vi "Get Full Tree.vi"(8 "error in (no error)":errorcluster, 11 "OpenHW in":refnum<class "OpenHW.lvclass">) -> (0 "error out":errorcluster, 2 "Full Tree":T1[](array[typedef]), 3 "OpenHW out":refnum<class "OpenHW.lvclass">)   [LabVIEW 2022 SP3, in "open-hw-mon-lv.lvlib" / "OpenHW.lvclass"]
uses:
  OpenHW.lvclass
  OpenHW.lvclass/OpenHW.ctl
  HW Node.ctl
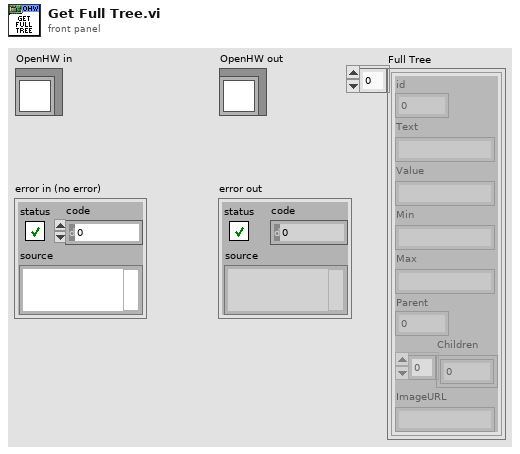
[diagram p1: front panel]
types:
  T1 = typedef "open-hw-mon-lv.lvlib/OpenHW.lvclass/HW Node.ctl" = cluster{"id":i32, "Text":string, "Value":string, "Min":string, "Max":string, "Parent":i32, "Children":i32[], "ImageURL":string}
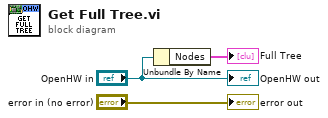
[diagram p0: block diagram]
diagram:
  n1 = Unbundle By Name("OpenHW in") -> ("Nodes"=→"Full Tree":T1[])
  "error out" <- "error in (no error)"
  "OpenHW out" <- "OpenHW in"
